vi "AlliGator Build Phasor Plot Image.vi"(7 "Display Range":cluster{"Slider 1":u32, "Slider 2":u32}, 8 "error in (no error)":errorcluster, 9 "Compute Phasor Plot (T)":bool=TRUE, 10 "Pixel Phasors Array (V x H)":csg[][](array[numeric]), 11 "Phasor Plot Image in":T2) -> (0 "error out":errorcluster, 1 "min value":u32, 2 "max value":u32, 3 "Phasor Plot Image out":T2)   [LabVIEW 2021, in "AlliGator Phasor Plot.lvlib"]
doc: "Builds Phasor Plot image based on phasor values and user-selected settings."
uses:
  AlliGator Phasor Plot.lvlib
  <vilib>/vision/Image Controls.llb/IMAQ Image.ctl
  Phasor/Phasor (g, s).ctl
  AlliGator Settings List.ctl
  AlliGator Variables List.ctl
  AlliGator Phasor Plot Reference Points.ctl
  bfe17851-1736-438a-bc86-f869e2daceed.vi
  Variant/Variant to Data/Variant to Boolean.vi
  AlliGator Globals, Variables & Constants.lvlib
  AlliGator Phasor Ratio.lvlib
  AlliGator Settings.lvlib
  Variant/Variant to Data/Variant to Data.lvlib
  Time/Time.lvlib
  Phasor/Phasor.lvlib
panel:
  out "Phasor of Max":T1
  out "min index(es)":i32[](array[numeric])
  out "max index(es)":i32[](array[numeric])
  out "min value SGL":sgl
  out "max value SGL":sgl
  out "elapsed (relative) seconds":dbl
  # "see the AlliGator License on the block diagram (Ctrl+E or Window:Show Block Diagram)"
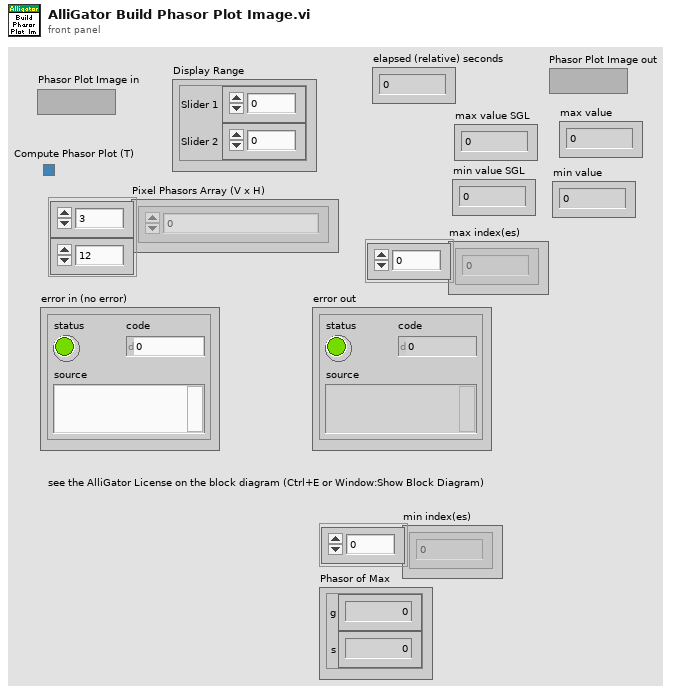
[diagram p1: front panel]
types:
  T1 = typedef "Phasor.lvlib/Phasor (g, s).ctl" = cluster{"g":dbl, "s":dbl}
  T2 = typedef "IMAQ Image.ctl" = refnum<image>
  T3 = typedef "AlliGator Settings.lvlib/AlliGator Settings List.ctl" = enum16{"GUI:Visible Settings Tab", "GUI:Last Run Version", "Source Image:Use Image Histogram for Contrast", "Source Image:Low Count Pixels Rejection Options", "Source Image:High Count Pixels Rejection Options", "Source Image:Use Image Brightness", "Source Image:Blend Overlay with Image Background", "Source Image:Use Fixed ROI Diameter", "Source Image:ROI Diameter", "Source Image:ROI Center Color", "Source Image:Peak Threshold", "Source Image:Intensity Threshold", "Source Image:Image Binning Options", "Source Image:Image Smoothing Options", "Source Image:Image Histogram Active", "Source Image:Invert Binary Mask", "Source Image:Hot Pixel Removal", "Source Image:Overlay Analyzed ROI Center", "Source Image:Auto-Adjust Contrast", "Source Image:Histogram Lower Percentile", "Source Image:Histogram Upper Percentile", "Source Image:Save Source Image", "Source Image:Scale Bar Options", "Source Image:Image Resolution (Pixel Size)", "Source Image:Flatfield Correction", "Data Information:Gate Width", "Data Information:Nanotime Gate Separation", "Data Information:Macrotime Gate Separation", "Data Information:Gate Step", "Data Information:# Gates", "Data Information:Gate Image Exposure", "Data Information:Gate Image Integration", "Data Information:Gates to Skip", "Data Information:Gates to Keep", "Data Information:Define Gates to", "Data Information:Channel Name", "Data Information:Available Channel Names", "Data Information:Channel Arithmetic", "Data Information:Background File Subtraction", "Data Information:Background File", "Data Information:Background Scaling Factor", "Data Information:Background Pile-up Correction", "Data Information:Background Pixel Well Capacity", "Data Information:Laser Period", "Data Information:SYNC Period", "Data Information:Pile-up Correction", "Data Information:Pixel Well Capacity", "Data Information:Dataset Scaling Factor", "Fluorescence Decay_Decay Pre-Processing:Reverse Gates", "Fluorescence Decay_Decay Pre-Processing:Verbose Decay Pre-Processing", "Fluorescence Decay_Decay Pre-Processing:Use Decay Pre-Processing", "Fluorescence Decay_Decay Pre-Processing:Background Subtraction", "Fluorescence Decay_Decay Pre-Processing:Background Definition Range", "Fluorescence Decay_Decay Pre-Processing:Baseline Subtraction Method", "Fluorescence Decay_Decay Pre-Processing:Operations Order", "Fluorescence Decay_Decay Pre-Processing:Smoothing Parameter", "Fluorescence Decay_Decay Pre-Processing:Shift Decay", "Fluorescence Decay_Decay Pre-Processing:Decay Shift Parameters", "Fluorescence Decay_Decay Pre-Processing:Fold Decay", "Fluorescence Decay_Decay Pre-Processing:# Folds", "Fluorescence Decay_Decay Pre-Processing:1-Normalize Decay", "Fluorescence Decay_Decay Pre-Processing:[0-1]-Normalize Decay", "Fluorescence Decay_Decay Pre-Processing:Smoothen Decay", "Fluorescence Decay_Decay Pre-Processing:Extrapolate Decay", "Fluorescence Decay_Decay Pre-Processing:Use Periodicity", "Fluorescence Decay_Decay Pre-Processing:Use Cursors", "Fluorescence Decay_Decay Pre-Processing:Tail Fraction", "Fluorescence Decay_Decay Pre-Processing:Head Fraction", "Fluorescence Decay_Decay Pre-Processing:Additional Points", "Fluorescence Decay_Decay Pre-Processing:Straighten Decay", "Fluorescence Decay_Decay Pre-Processing:Constant Background", "Fluorescence Decay_Decay Pre-Processing:Pixel-Normalize Decay", "Fluorescence Decay_Advanced Analysis:Extract IRF instead of Decay", "Fluorescence Decay_Advanced Analysis:IRF Extraction Options", "Fluorescence Decay_Advanced Analysis:IRF Optimization Options", "Fluorescence Decay_Advanced Analysis:Square Pulse Options", "Fluorescence Decay_Advanced Analysis:IRF Order", "Fluorescence Decay_Advanced Analysis:IRF Time Constants", "Fluorescence Decay_Advanced Analysis:Wavelet Analysis Options", "Fluorescence Decay_Advanced Analysis:Average Lifetime Options", "Fluorescence Decay_Fit Options:Fit Options", "Fluorescence Decay_Fit Options:Use Legacy Fitting Approach", "Fluorescence Decay_Fit Options:Use Data Information Laser Period", "Fluorescence Decay_Fit Parameters:Displayed Fit Parameters", "Fluorescence Decay_Fit Parameters:Fit Parameter Constraints", "Fluorescence Decay_Fit Parameters:Export Tabulated Results", "Fluorescence Decay_Fit Parameters:MLE Baseline Offset Type", "Fluorescence Decay_Fit Parameters:MLE Baseline Offset", "Fluorescence Decay_Fit Parameters:Guess Parameter Names", "Fluorescence Decay_Fit Parameters:Guess Parameter Values", "Fluorescence Decay_Fit Parameters:Guess Parameters Options", "Fluorescence Decay_Styles:Show Last Decay Only", "Fluorescence Decay_Styles:Decay Graph Color Array", "Fluorescence Decay:Decay Graph Active", "Fluorescence Decay Statistics:Min Peak Value", "Fluorescence Decay Statistics:Reject Low Decay Peak Pixels", "Fluorescence Decay Statistics:Reject High Decay Peak Pixels", "Fluorescence Decay Statistics:Max Peak Value", "Time Traces:Use File Timestamp", "Time Traces:Time Step", "Time Traces:Use Intensity Correction File", "Time Traces:Intensity Correction File", "Phasor Plot:Phasor Plot Smoothing Options", "Phasor Plot:Phasor Plot Size", "Phasor Plot:Phasor Plot Graphics Options", "Phasor Plot:Cumulative Phasor Plot", "Phasor Plot:Use Phasor Brightness", "Phasor Plot:Blend Overlay with Phasor Background", "Phasor Plot:Save Phasor Plot", "Phasor Plot:Show References", "Phasor Plot:Phasor Ratio Decay Range", "Phasor Plot:Exponential Fading", "Phasor Plot:Phasor Ratio Reference Colors", "Phasor Plot:Reference Radius", "Phasor Plot:Show Color Map Vertices", "Phasor Plot:Phasor Plot Active", "Phasor Plot:Phasor Ratio Color Map Type", "Phasor Plot:Phasor Ratio Color Map", "Phasor Plot:Phasor Ratio Display Range", "Phasor Plot:Selected Image ROI(s)", "Phasor Plot:All Image ROIs", "Phasor Plot:Selected Phasor Plot ROI(s)", "Phasor Plot:All Phasor Plot ROIs", "Phasor Plot:Phasor Ratio Color-Coded Quantity", "Phasor Plot:Store Phasor Harmonics", "Phasor Plot:Draw Reference Segment", "Phasor Plot:User-Defined Quantity", "Phasor Graph:Phasor Frequency", "Phasor Graph:Phasor Ratio Type", "Phasor Graph:Pixel-level Phasor Computation", "Phasor Graph:Save Phasor Graph", "Phasor Graph:Phasor Graph Active", "Phasor Graph:Phasor SDV Options", "Phasor Calibration:Use Backup Calibration if needed", "Phasor Graph:Define Shortest Lifetime as", "Phasor Calibration:Backup Calibration Type", "Phasor Calibration:Calibration Type", "Phasor Calibration:Calibration Lifetime", "Phasor Calibration:Calibration Map Algorithm", "Single-Exponential Phasor Locus (SEPL):Gate Parameters", "Single-Exponential Phasor Locus (SEPL):User-defined Gate", "Single-Exponential Phasor Locus (SEPL):User-defined IRF", "Single-Exponential Phasor Locus (SEPL):Phasor Parameters", "Single-Exponential Phasor Locus (SEPL):Decay & IRF Parameters", "Single-Exponential Phasor Locus (SEPL):Display Parameters", "Lifetime Analysis:Decay Analysis Parameters", "Lifetime Analysis:Lifetime Map Active", "Plugins:Python Settings", "Miscellaneous:Verbose Mode", "Miscellaneous:Beep after Script", "Miscellaneous:Saved Image File Format", "Miscellaneous:Exported Gate Image Settings", "Miscellaneous:Include Loading in Timing", "Miscellaneous:Verbose Settings Mode", "Miscellaneous:Histogram Options", "Miscellaneous:Beep on Error", "Miscellaneous:# Logical Processors Used", "Miscellaneous:ROI Description Max Characters", "Miscellaneous:Verbose Error Mode", "Miscellaneous:Transparent Mask Color"}
  T4 = typedef "AlliGator Globals, Variables & Constants.lvlib/AlliGator Variables List.ctl" = enum16{"---- GUI ----", "Initialization Status", "State Indicators Refnum", "Original AlliGator Menu Items", "Current Action Loop State", "Script in progress", "Playback", "Loop Playback", "Search ROI Used", "Search ROI", "Decay Graph Max Legend Size", "Intensity Graph Max Legend Size", "Decay Statistics Graph Max Legend Size", "Phasor Graph Max Legend Size", "Phasor Ratio Graph Max Legend Size", "Lifetime Graph Max Legend Size", "---- Files ----", "Export Dataset Frames as Individual Files", "Show Batch Export Help Balloons", "Frames in Dataset", "ptu File Frame Start Indices", "Current Frame in Dataset", "Current Frame Timestamp", "------ Python Plugins ------", "Python Plugins Information", "Python Session", "Valid Python Session?", "---- Source Image ----", "Dataset Loaded", "Dataset Metadata", "Dataset Channel", "Dataset Data Description", "Background Dataset Metadata", "Background Dataset Channel", "Background Dataset Data Description", "Background File Subtraction", "Background File Path", "Background File Pile-up Correction", "Background File Pixel Well Capacity", "Background File Scaling Factor", "Source Image ROIs", "Current Source Image ROI", "Source Image ROI Event Refnum", "X_Source Image Display Range", "X_Source Image Palette Information", "Source Image Palette List", "Source Image Scale", "Current Dataset Load Settings", "Source Image:ROI Overlay Color", "---- Image Profile Window ----", "Image Profile:Overlay ROI in Source Image", "Image Profile Window Event Refnum", "Image Profile:IntensityType", "Image Profile:Intensity Average Type", "Image Profile:Intensity-weighted SDV", "Image Profile:Box Profile Type", "Image Profile Window Open", "Image Profile:Plotted Fit Parameter", "X_Type of Displayed Image", "X_Time Gate Slider", "Dataset Path", "Source Image Overlay to Erase", "Is Displayed Image Accumulated", "White Light Image Modified", "Mask Image Modified", "Macrotime Gate Separation", "------ Phasor Graph -------", "Phasor Graph:Show Line", "---- Phasor Plot ---", "Phasor Plot Parameters Changed", "FLI Dataset Modified since last Phasor Plot Calculation", "Phasor Harmonics Data", "Selected Phasor Harmonics", "Phasor Harmonic Manager Event Refnum", "Phasor Plot ROIs", "Current Phasor Plot ROI", "Phasor Plot ROI Event Refnum", "Phasor Plot Image Reference Points", "Phasor Plot Computed", "Phasor Plot Palette Information", "Phasor Plot Palette List", "Phasor Ratio Palette Information", "Phasor Ratio Palette List", "Phasor Image Scale", "Phasor Plot Image Overlay to Erase", "Phasor Plot Image Elements to Update", "Current Phasor Plot Calculation Parameters", "Current Phasor Calibration Options", "Reset Cumulated Phasor Plot", "Phasor Ratio Reference 1", "Phasor Ratio Lifetime Reference 1", "Phasor Ratio Reference 1 Frequency", "Phasor Ratio Reference 2", "Phasor Ratio Lifetime Reference 2", "Phasor Ratio Reference 2 Frequency", "---- Decay Analysis ----", "Number of Selected Decays to Fit", "LS Fit Results", "LAR Fit Results", "BS Fit Results", "Last Decay Max - Min", "Best Fit Parameters", "Best Fit Parameter Names", "Actual Size X", "Actual Size Y", "Binning X", "Binning Y", "Actual # Gates", "Dataset Number", "Gates to...", "Gates Skipped", "Gates to keep", "Gate Step", "Gate Separation", "Reversed Gates", "Pile-up Correction", "Pixel Well Capacity", "Background Subtracted", "Background Subtraction Method", "Background Definition Range", "Background File (deprecated)", "Number of Dataset Accumulated", "Array of Accumulated Dataset Paths", "Do Averaged Datasets", "Destination File Path", "Process Plot Target", "Use 1/D as Phasor Frequency", "---- Decay Fit Parameter Map -----", "Decay Fit Parameter Map Palette Information", "Decay Fit Parameter Map Palette List", "Local Decay Graph Window Event Refnum", "------- Local Decay Window ---------", "Use normalized IRF for convolution", "----- Miscellaneous ----", "Skippable Dialog Windows Status"}
  T5 = typedef "AlliGator Phasor Ratio.lvlib/AlliGator Phasor Plot Reference Points.ctl" = cluster{"O_h":dbl, "O_v":dbl, "1_h":dbl, "1_v":dbl}
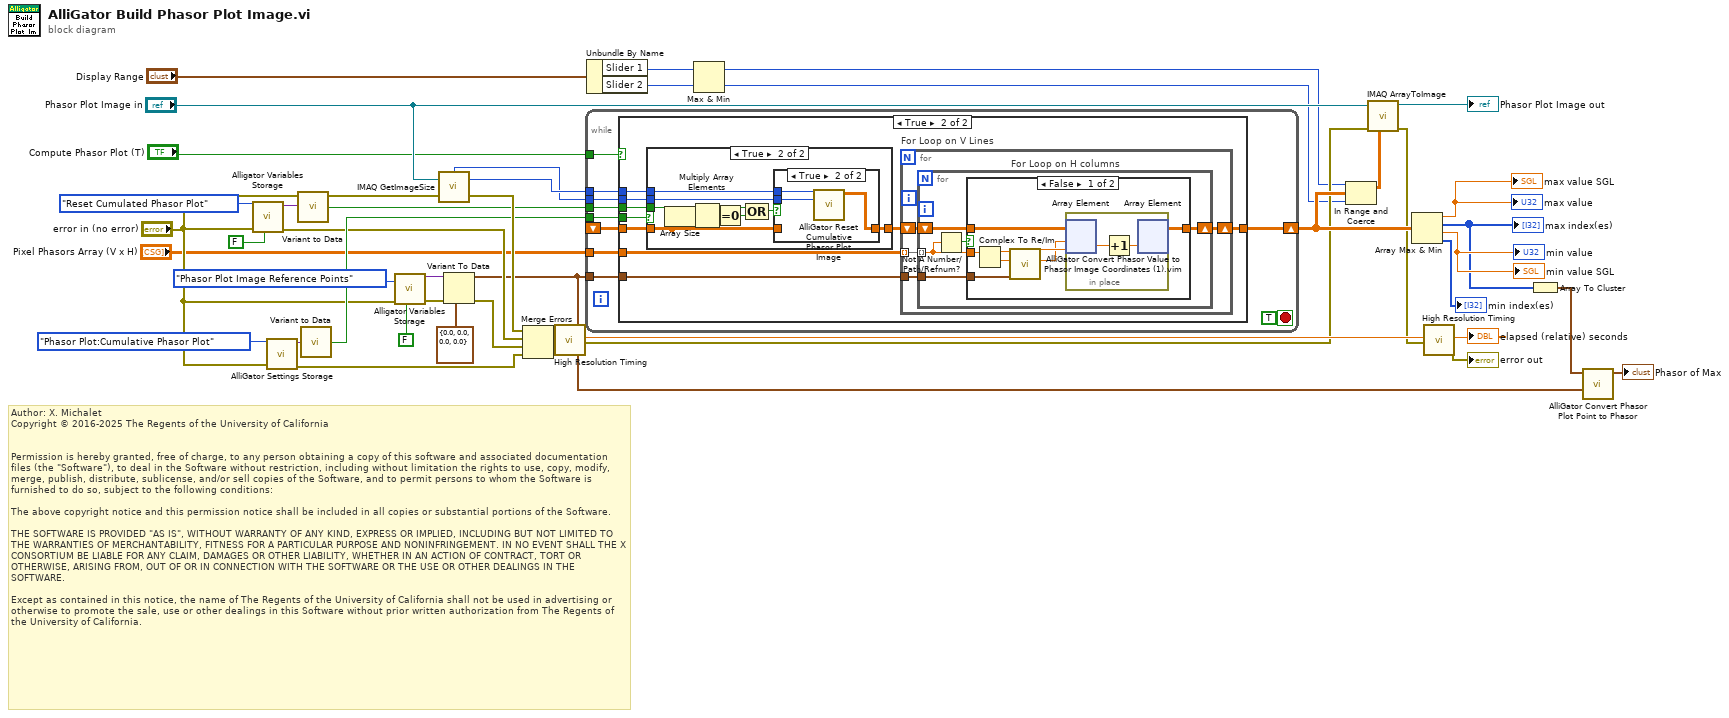
[diagram p0: block diagram]
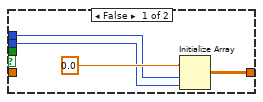
[diagram p3: hidden frame]
diagram:
  # "Author: X. Michalet\nCopyright © 2016-2025 The Regents of the University of California\n \n\nPermission is hereby granted, free of charge, to any person obtaining a copy of this software and associated documentation files (the \"Software\"), to deal in the Software without restriction, including without limitation the rights to use, copy, modify, merge, publish, distribute, sublicense, and/or sell copies of the Software, and to permit persons to whom the Software is furnished to do so, subject to the following conditions:\n\nThe above copyright notice and this permission notice shall be included in all copies or substantial portions of the Software.\n\nTHE SOFTWARE IS PROVIDED \"AS IS\", WITHOUT WARRANTY OF ANY KIND, EXPRESS OR IMPLIED, INCLUDING BUT NOT LIMITED TO THE WARRANTIES OF MERCHANTABILITY, FITNESS FOR A PARTICULAR PURPOSE AND NONINFRINGEMENT. IN NO EVENT SHALL THE X CONSORTIUM BE LIABLE FOR ANY CLAIM, DAMAGES OR OTHER LIABILITY, WHETHER IN AN ACTION OF CONTRACT, TORT OR OTHERWISE, ARISING FROM, OUT OF OR IN CONNECTION WITH THE SOFTWARE OR THE USE OR OTHER DEALINGS IN THE SOFTWARE.\n\nExcept as contained in this notice, the name of The Regents of the University of California shall not be used in advertising or otherwise to promote the sale, use or other dealings in this Software without prior written authorization from The Regents of the University of California."
  n1 = call "Alligator Variables Storage.vi"("Get(F)/Set"=FALSE, "AlliGator Variable"=AlliGator_Variables_List."Reset Cumulated Phasor Plot" ("Alligator Variable"), "Error In"="error in (no error)") -> ("Error Out"=w22:errorcluster, "Data out"=w32:variant)  [unwired: 6 in, 1 out]
  n2 = call "AlliGator Settings Storage.vi"("AlliGator Settings List"=AlliGator_Settings_List."Phasor Plot:Cumulative Phasor Plot", "Error In"="error in (no error)") -> ("Error Out"=w20:errorcluster, "Variant Data out"=w27:variant)  [unwired: 8 in]
  n3 = call-poly "Variant to Data.vi"("Variant"=w32) -> ("Value"=w29:bool)  [unwired: 8 in]
  n4 = call-poly "Variant to Data.vi"("Variant"=w27) -> ("Value"=w35:bool)  [unwired: 8 in]
  n5 = call "Alligator Variables Storage.vi"("Get(F)/Set"=FALSE, "AlliGator Variable"=AlliGator_Variables_List."Phasor Plot Image Reference Points" ("Alligator Variable"), "Error In"="error in (no error)") -> ("Error Out"=w41:errorcluster, "Data out"=w43:variant)  [unwired: 6 in, 1 out]
  n6 = call "IMAQ GetImageSize"("Image"="Phasor Plot Image in", "error in (no error)"="error in (no error)") -> ("Y Resolution"=w13:i32, "X Resolution"=w12:i32, "error out"=w40:errorcluster)  [unwired: 2 in]
  n7 = Variant To Data(error in=w41, type=T5 {"O_h"=0.0, "O_v"=0.0, "1_h"=0.0, "1_v"=0.0} ("Phasor Plot Reference Points"), Variant=w43) -> (data=w9:T5, error out=w21:errorcluster)
  n8 = Merge Errors(w40, w22, w21, w20) -> (w23:errorcluster)
  n9 = call "High Resolution Timing.vi"("Error In"=w23) -> ("elapsed (relative) seconds"=w26:dbl, "Error Out"=w17:errorcluster)  [unwired: 16 in, 1 out]
  n10 = while {
    tunnel: "Pixel Phasors Array (V x H)" -> [w53]
    tunnel: w9 -> [w52]
    tunnel: w13 -> [w50]
    tunnel: w12 -> [w49]
    shift-right: [w51] -> w19
    shift-left: _ -> [w47]
    tunnel: w35 -> [w48]
    tunnel: w29 -> [w45]
    tunnel: "Compute Phasor Plot (T)" -> [w44]
    stop <- TRUE stop-if-true
    n11 = case shown="True" w44 {
      tunnel: w53 -> [_ w63]
      tunnel: w52 -> [_ w62]
      tunnel: [w54 w60] -> w51
      tunnel: w50 -> [_ w59]
      tunnel: w49 -> [_ w58]
      tunnel: w48 -> [_ w57]
      tunnel: w47 -> [w54 w56]
      tunnel: w45 -> [_ w55]
      frame False {
      }
      frame True {
        n12 = case shown="True" w57 {
          tunnel: [w67 w75] -> w61
          tunnel: w59 -> [w65 w74]
          tunnel: w58 -> [w64 w73]
          tunnel: w56 -> [_ w72]
          tunnel: w55 -> [_ w76]
          frame False {
            n13 = Initialize Array(sgl 0.0, w65, w64) -> (w67:sgl[][])
          }
          frame True {
            n14 = Array Size(array=w72) -> (size(s)=w71:i32[])
            n15 = Multiply Array Elements(1:w71) -> (0:w70:i32)
            n16 = Equal To 0?(x=w70) -> (x = 0?=w68:bool)
            n17 = Compound Arithmetic op=OR(w76, w68) -> (w69:bool)
            n18 = case shown="True" w69 {
              tunnel: w72 -> [w77 _]
              tunnel: [w77 w78] -> w75
              tunnel: w74 -> [_ w80]
              tunnel: w73 -> [_ w79]
              frame False {
              }
              frame True {
                n19 = call "AlliGator Reset Cumulative Phasor Plot Image.vi"("X Resolution"=w79, "Y Resolution"=w80) -> ("Array"=w78:sgl[][])  [unwired: 9 in]
              }
            }
          }
        }
        n20 = for "For Loop on V Lines" {
          tunnel: w63 -> [w84] mode=indexing
          tunnel: w62 -> [w83]
          shift-right: [w81] -> w60
          shift-left: w61 -> [w82]
          n21 = for "For Loop on H columns" {
            tunnel: w84 -> [w86] mode=indexing
            tunnel: w83 -> [w89]
            shift-right: [w87] -> w81
            shift-left: w82 -> [w88]
            n22 = Not A Number/Path/Refnum?(number/path/refnum=w86) -> (NaN/Path/Refnum?=w85:bool)
            n23 = case shown="False" w85 {
              tunnel: w89 -> [w97 _]
              tunnel: w88 -> [w94 w100]
              tunnel: [w93 w100] -> w87
              tunnel: w86 -> [w90 _]
              frame False {
                n24 = Complex To Re/Im(x + iy=w90) -> (x=w96:sgl, y=w95:sgl)
                n25 = call "AlliGator Convert Phasor Value to Phasor Image Coordinates (1).vim"("Phasor Plot Reference Points"=w97, "Phasor s"=w95, "Phasor g"=w96) -> ("Phasor Plot y"=w91:dbl, "Phasor Plot x"=w92:dbl)  [unwired: 7 in]
                n26 = in-place {
                  n27 = in-place-array #1(w94, w91, w92) -> (w99:sgl)
                  n28 = Increment(x=w99) -> (x+1=w98:sgl)
                  n29 = in-place-array #1(w98) -> (w93:sgl[][])  [unwired: 2 out]
                }
              }
              frame True {
              }
            }
          }
        }
      }
    }
  }
  n30 = Unbundle By Name("Display Range") -> ("Slider 1"=w4:u32, "Slider 2"=w3:u32)
  n31 = Max & Min(x=w4, y=w3) -> (max(x,y)=w2:u32, min(x,y)=w1:u32)
  n32 = In Range and Coerce(upper limit=w2, x=w19, lower limit=w1) -> (coerced(x)=w18:sgl[][])  [unwired: 1 out]
  n33 = call "IMAQ ArrayToImage"("Image Pixels (Float)"=w18, "error in (no error)"=w17, "Image"="Phasor Plot Image in") -> ("error out"=w16:errorcluster, "Image Out"=→"Phasor Plot Image out":T2)  [unwired: 7 in]
  n34 = Array Max & Min(array=w19) -> (max value=→"max value" →"max value SGL":sgl, max index (indices)=w8:i32[], min value=→"min value" →"min value SGL":sgl, min index (indices)=→"min index(es)":i32[])
  "max index(es)" <- w8
  n35 = call "High Resolution Timing.vi"("relative seconds (NaN)"=w26, "Error In"=w16) -> ("elapsed (relative) seconds"=→"elapsed (relative) seconds":dbl, "Error Out"=→"error out":errorcluster)  [unwired: 15 in, 1 out]
  n36 = Array To Cluster(array=w8) -> (cluster=w7:cluster{"[0]":i32, "[1]":i32})
  n37 = call "AlliGator Convert Phasor Plot Point to Phasor.vi"("Phasor Plot Reference Points"=w9, "Phasor Plot Point"=w7) -> ("Phasor"=→"Phasor of Max":T1)  [unwired: 9 in]
